vi "dropCols.vi"(11 "data":dbl[][](array[numeric])) -> (3 "data (columns dropped)":dbl[][](array[numeric]))   [LabVIEW 2014]
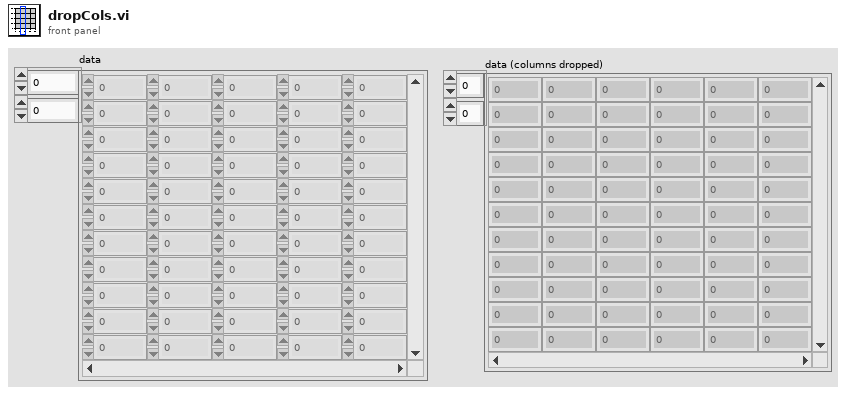
[diagram p1: front panel]
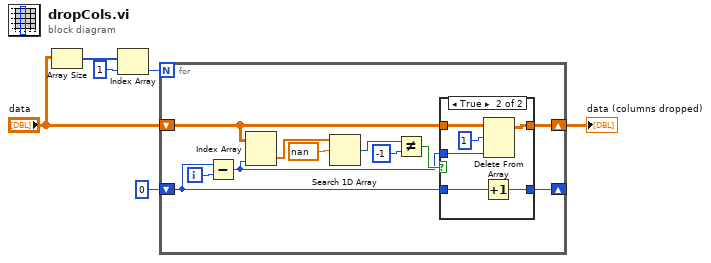
[diagram p0: block diagram]
diagram:
  n1 = Array Size(array="data") -> (size(s)=w5:i32[])
  n2 = Index Array(array=w5, index=1) -> (element=w4:i32)
  n3 = for {
    N: w4 -> [_]
    shift-right: [w10] -> w1
    shift-left: "data" -> [w11]
    shift-right: [w7] -> _
    shift-left: 0 -> [w8]
    i -> [w17]
    n4 = Subtract(x=w8, y=w17) -> (x-y=w9:i32)
    n5 = Index Array(array=w11, index (col)=w9) -> (element=w16:dbl[])  [unwired: 1 in]
    n6 = Search 1D Array(1D array=w16, element=nan) -> (index of element=w14:i32)  [unwired: 1 in]
    n7 = Not Equal?(x=w14, y=-1) -> (x != y?=w12:bool)
    n8 = case shown="True" w12 {
      tunnel: w11 -> [w19 w25]
      tunnel: [w19 w22] -> w10
      tunnel: w9 -> [_ w24]
      tunnel: w8 -> [w18 w21]
      tunnel: [w18 w20] -> w7
      frame False {
      }
      frame True {
        n9 = Increment(x=w21) -> (x+1=w20:i32)
        n10 = Delete From Array(array=w25, length=1, index (col)=w24) -> (array with subset deleted=w22:dbl[][])  [unwired: 1 in, 1 out]
      }
    }
  }
  "data (columns dropped)" <- w1
